vi "画直线.vi"(10 "Straight Edge (底边)":T1, 11 "引用句柄输入":T2) -> ()   [LabVIEW 2014]
uses:
  <vilib>/vision/Image Controls.llb/IMAQ Image.ctl
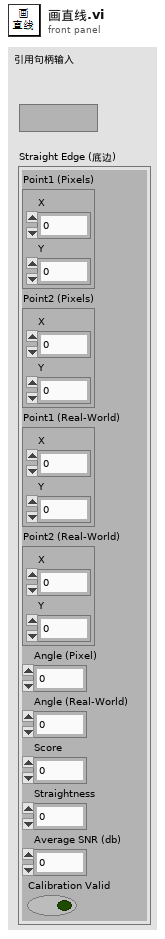
[diagram p1: front panel]
types:
  T1 = cluster{"Point1 (Pixels)":cluster{"X":sgl, "Y":sgl}, "Point2 (Pixels)":cluster{"X":sgl, "Y":sgl}, "Point1 (Real-World)":cluster{"X":sgl, "Y":sgl}, "Point2 (Real-World)":cluster{"X":sgl, "Y":sgl}, "Angle (Pixel)":dbl, "Angle (Real-World)":dbl, "Score":dbl, "Straightness":dbl, "Average SNR (db)":dbl, "Calibration Valid":bool}
  T2 = typedef "IMAQ Image.ctl" = refnum<image>
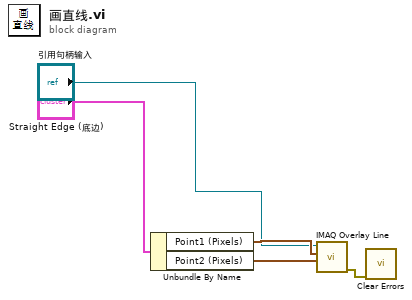
[diagram p0: block diagram]
diagram:
  n1 = Unbundle By Name("Straight Edge (底边)") -> ("Point1 (Pixels)"=w3:cluster{"X":sgl, "Y":sgl}, "Point2 (Pixels)"=w4:cluster{"X":sgl, "Y":sgl})
  n2 = call "IMAQ Overlay Line"("End Point"=w4, "Start Point"=w3, "Image"="引用句柄输入") -> ("error out"=w5:errorcluster)  [unwired: 7 in, 1 out]
  n3 = call <vilib>:"Clear Errors.vi"("error in (no error)"=w5) -> ()  [unwired: 5 in, 2 out]
